vi "BATT DATA.vi"(0 "BATTERY EMULATOR":T1) -> (14 "MODEL SELECTION":dbl, 15 "CONTROL SELECTION":dbl, 16 "VOLTAGE":dbl, 17 "CURRENT":dbl, 18 "POWER":dbl)   [LabVIEW 2025]
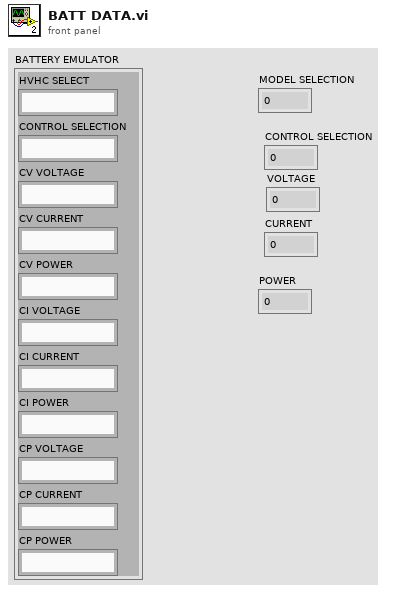
[diagram p1: front panel]
types:
  T1 = cluster{"HVHC SELECT":string, "CONTROL SELECTION":string, "CV VOLTAGE":string, "CV CURRENT":string, "CV POWER":string, "CI VOLTAGE":string, "CI CURRENT":string, "CI POWER":string, "CP VOLTAGE":string, "CP CURRENT":string, "CP POWER":string}
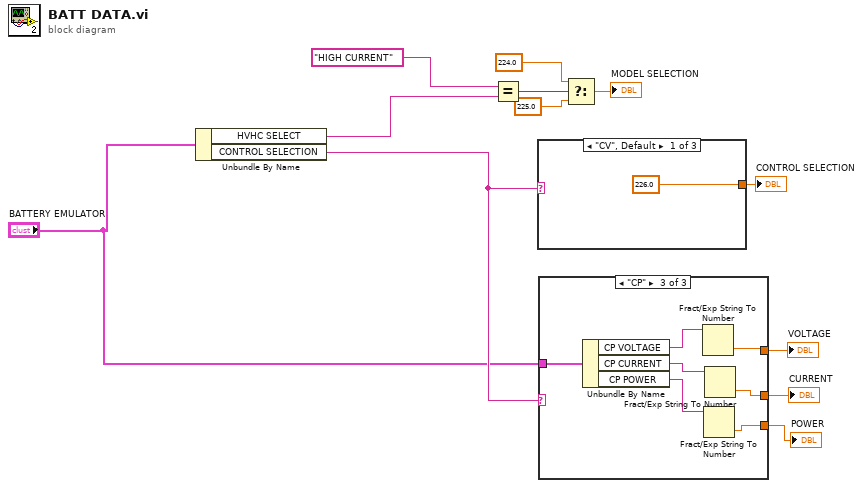
[diagram p0: block diagram]
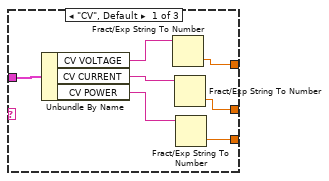
[diagram p2: hidden frame]
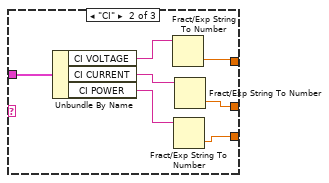
[diagram p3: hidden frame]
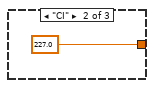
[diagram p4: hidden frame]
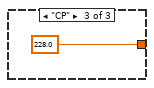
[diagram p5: hidden frame]
diagram:
  n1 = Unbundle By Name("BATTERY EMULATOR") -> ("HVHC SELECT"=w12:string, "CONTROL SELECTION"=w6:string)
  n2 = Equal?(x="HIGH CURRENT" ("y"), y=w12) -> (x = y?=w10:bool)
  n3 = case shown="\"CV\", Default" w6 {
    tunnel: [226.0 227.0 228.0] -> w7
    frame "CV", Default {
    }
    frame "CI" {
    }
    frame "CP" {
    }
  }
  "CONTROL SELECTION" <- w7
  n4 = case shown="\"CP\"" w6 {
    tunnel: "BATTERY EMULATOR" -> [w22 w29 w36]
    tunnel: [w18 w27 w34] -> w4
    tunnel: [w17 w25 w32] -> w3
    tunnel: [w16 w23 w30] -> w2
    frame "CV", Default {
      n5 = Unbundle By Name(w22) -> ("CV VOLTAGE"=w21:string, "CV CURRENT"=w20:string, "CV POWER"=w19:string)
      n6 = Fract/Exp String To Number(string=w21) -> (number=w18:dbl)  [unwired: 3 in, 1 out]
      n7 = Fract/Exp String To Number(string=w20) -> (number=w17:dbl)  [unwired: 3 in, 1 out]
      n8 = Fract/Exp String To Number(string=w19) -> (number=w16:dbl)  [unwired: 3 in, 1 out]
    }
    frame "CI" {
      n9 = Unbundle By Name(w29) -> ("CI VOLTAGE"=w28:string, "CI CURRENT"=w26:string, "CI POWER"=w24:string)
      n10 = Fract/Exp String To Number(string=w28) -> (number=w27:dbl)  [unwired: 3 in, 1 out]
      n11 = Fract/Exp String To Number(string=w24) -> (number=w23:dbl)  [unwired: 3 in, 1 out]
      n12 = Fract/Exp String To Number(string=w26) -> (number=w25:dbl)  [unwired: 3 in, 1 out]
    }
    frame "CP" {
      n13 = Unbundle By Name(w36) -> ("CP VOLTAGE"=w35:string, "CP CURRENT"=w33:string, "CP POWER"=w31:string)
      n14 = Fract/Exp String To Number(string=w35) -> (number=w34:dbl)  [unwired: 3 in, 1 out]
      n15 = Fract/Exp String To Number(string=w31) -> (number=w30:dbl)  [unwired: 3 in, 1 out]
      n16 = Fract/Exp String To Number(string=w33) -> (number=w32:dbl)  [unwired: 3 in, 1 out]
    }
  }
  "VOLTAGE" <- w4
  "CURRENT" <- w3
  "POWER" <- w2
  n17 = Select(t=224.0, s=w10, f=225.0) -> (s? t:f=→"MODEL SELECTION":dbl)
